vi "CNT Init Counter.vi"(7 "pInitConfig":T1, 8 "error in (no error)":errorcluster, 9 "Channel":u8, 10 "DevIndex":i32, 11 "DevType":i32) -> (0 "error out":errorcluster, 3 "function return":i32)   [LabVIEW 2012, in "ControlCNT.lvlib"]
doc: "int WINAPI CNT_InitCounter(int DevType, int DevIndex, unsigned char Channel, PCNT_INIT_CONFIG pInitConfig);"
uses:
  ControlCNT.lvlib
  Ginkgo_Driver.dll
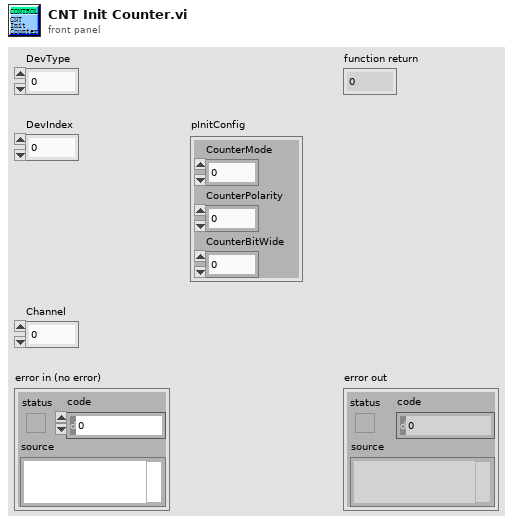
[diagram p1: front panel]
types:
  T1 = cluster{"CounterMode":u8, "CounterPolarity":u8, "CounterBitWide":u8}
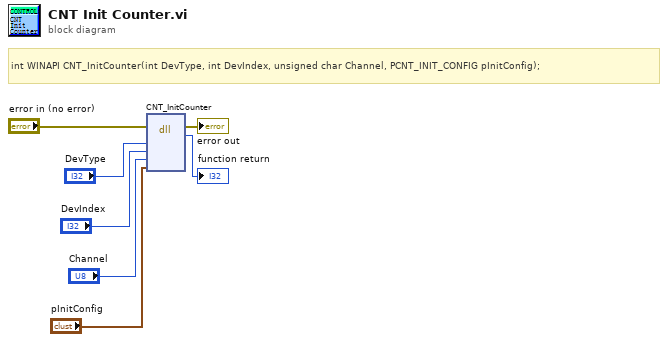
[diagram p0: block diagram]
diagram:
  # "int WINAPI CNT_InitCounter(int DevType, int DevIndex, unsigned char Channel, PCNT_INIT_CONFIG pInitConfig);"
  n1 = dll-call lib="E:/Project/vt_ginkgo/truck/Ginkgo Driver/vs2010/Ginkgo_USB-I2C_API_v2.0.3.0/lib/labview_64bit/ControlCNT/Ginkgo_Driver.*" fn="CNT_InitCounter"(error in="error in (no error)", "DevType"="DevType", "DevIndex"="DevIndex", "Channel"="Channel", "pInitConfig"="pInitConfig") -> (error out=→"error out":errorcluster, →"function return":i32)  [unwired: 6 in, 1 out]
